vi "Robo Team Globals.vi"() -> ()   [LabVIEW 2015]
uses:
  Robo Team Engine Command.ctl
  Robo Axis Ref.ctl
  Robo System State Refs.ctl
  RT Controls/Generic instruction typedef.ctl
  IP Dev Area/IP results.ctl
panel:
  out "IP Results":T1
  in  "Update Pos":bool
  out "CMD time":timestamp
  in  "CmdWriter":refnum<k21>
  in  "In Action":bool
  in  "Sys State Refs":T2
  in  "EM Stop":bool
  out "Axis Refs":T3
  out "Stream Engine Q":refnum<queue>
  out "Stream Engine Not":refnum<notifier>
  out "Top Q":refnum<queue>
  out "Top Not":refnum<notifier>
  out "Front Q":refnum<queue>
  out "Front Not":refnum<notifier>
  out "Side Q":refnum<queue>
  out "Side Not":refnum<notifier>
  out "Engine Q":refnum<queue>
  out "Engine Not":refnum<notifier>
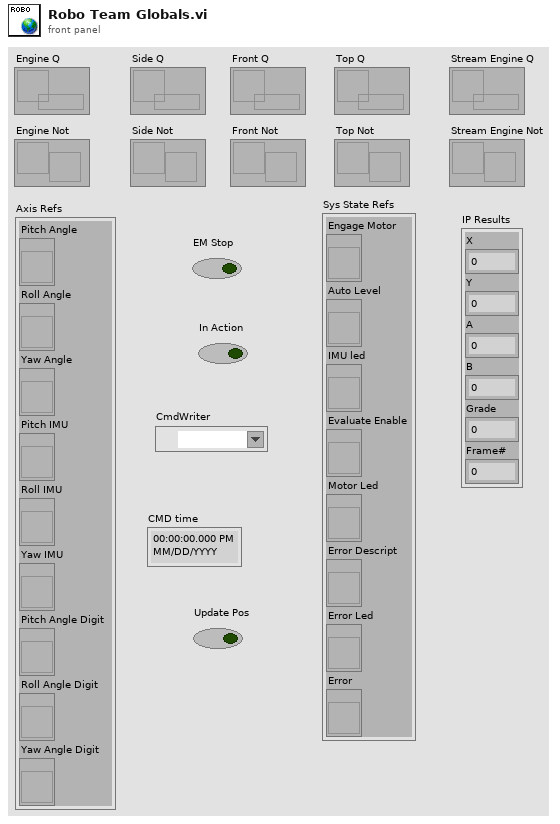
[diagram p1: front panel]
types:
  T1 = typedef "IP results.ctl" = cluster{"X":u16, "Y":u16, "A":dbl, "B":dbl, "Grade":u16, "Frame#":u16}
  T2 = typedef "Robo System State Refs.ctl" = cluster{"Engage Motor":refnum<vi>, "Auto Level":refnum<vi>, "IMU led":refnum<vi>, "Evaluate Enable":refnum<vi>, "Motor Led":refnum<vi>, "Error Descript":refnum<vi>, "Error Led":refnum<vi>, "Error":refnum<vi>}
  T3 = typedef "Robo Axis Ref.ctl" = cluster{"Pitch Angle":refnum<vi>, "Roll Angle":refnum<vi>, "Yaw Angle":refnum<vi>, "Pitch IMU":refnum<vi>, "Roll IMU":refnum<vi>, "Yaw IMU":refnum<vi>, "Pitch Angle Digit":refnum<vi>, "Roll Angle Digit":refnum<vi>, "Yaw Angle Digit":refnum<vi>}
diagram:
